vi "get_voltage_and_current.vi"(8 "error in":errorcluster, 11 "VISA resource name":refnum<visa-resource-name>="COM1") -> (0 "error out":errorcluster, 3 "Response":string)   [LabVIEW 2020]
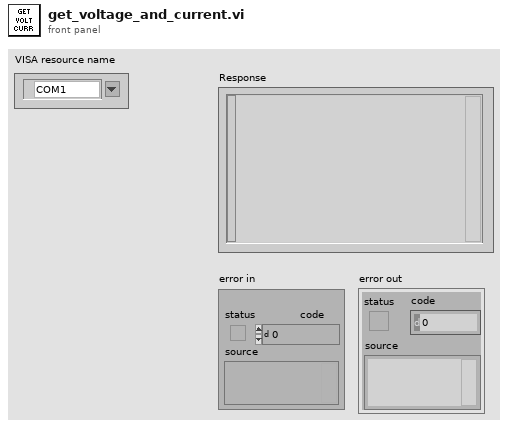
[diagram p1: front panel]
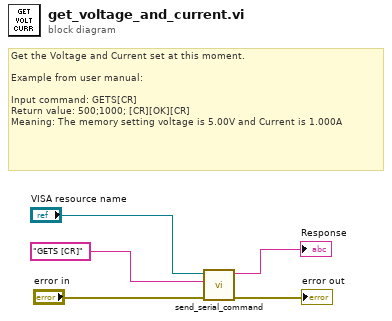
[diagram p0: block diagram]
diagram:
  # "Get the Voltage and Current set at this moment.\n\nExample from user manual:\n\nInput command: GETS[CR]\nReturn value: 500;1000; [CR][OK][CR]\nMeaning: The memory setting voltage is 5.00V and Current is 1.000A"
  n1 = call "send_serial_command.vi"("error in (no error)"="error in", "Command"="GETS [CR]", "VISA resource name"="VISA resource name") -> ("error out"=→"error out":errorcluster, "Response"=→"Response":string)  [unwired: 7 in]
